vi "Dual_image_synced.vi"() -> ()   [LabVIEW 2013]
uses:
  <vilib>/DAQmx/create/channels.llb/DAQmx Create Channel (CO-Pulse Generation-Frequency).vi
  <vilib>/DAQmx/configure/timing.llb/DAQmx Timing (Implicit).vi
  <vilib>/vision/driver/NI_Vision_Acquisition_Software.lvlib
  <resource>/objmgr/imaqdx.rc
  <resource>/objmgr/daqmx.rc
panel:
  in  "Gain 2":dbl(slide)=575.0 min=350.0 max=1000.0 step=1.0 scale=350.0..1000.0
  in  "VR2":dbl(slide)=65.0 min=0.0 max=255.0 step=1.0 scale=0.0..255.0
  in  "VR1":dbl(slide)=60.0 min=0.0 max=255.0 step=1.0 scale=0.0..255.0
  in  "UB2":dbl(slide)=160.0 min=0.0 max=255.0 step=1.0 scale=0.0..255.0
  in  "UB1":dbl(slide)=165.0 min=0.0 max=255.0 step=1.0 scale=0.0..255.0
  in  "Shutter":dbl(slide)=4095.0 min=0.0 max=4095.0 step=1.0 scale=4.095..4095.0 scale format="%#.0f"
  in  "Brightness":dbl(slide)=100.0 min=0.0 max=255.0 step=1.0 scale=0.0..255.0
  in  "Gain":dbl(slide)=600.0 min=350.0 max=1000.0 step=1.0 scale=350.0..1000.0
  in  "Test Description":string="test"
  in  "Storage Directory":path=path "C:/Users/Regen/Desktop/Users/Ryan Gergely/3D_DIC"
  out "Image 2":T1(plugin-control)
  out "Buffer Number 2":u32
  out "Frame Rate 2":dbl
  in  "Camera Name 2":refnum<k21>="cam2" caption="IMAQdx Session"
  in  "Pule Frequency":dbl=2.0 format="%.1f"
  out "Actual Duty Cycle":dbl
  out "Actual Pulse Frequency":dbl
  in  "Stop":bool
  in  "Start Trigger Mode":bool
  out "Frame Rate 1":dbl
  out "Buffer Number 1":u32
  in  "Camera Name 1":refnum<k21>="cam1" caption="IMAQdx Session"
  out "Image":T1(plugin-control)
  # "1) Set Test Description and Storage Directory"
  # "2) Select Cameras"
  # "3) Start VI"
  # "4) Set Frequency and Exposure and White Balance\n(Before Start Trigger)"
  # "5)"
  # "6) Stop When Done"
  # "Exposure Settings - Both Cameras"
  # "White Balance - Camera1"
  # "White Balance - Camera2"
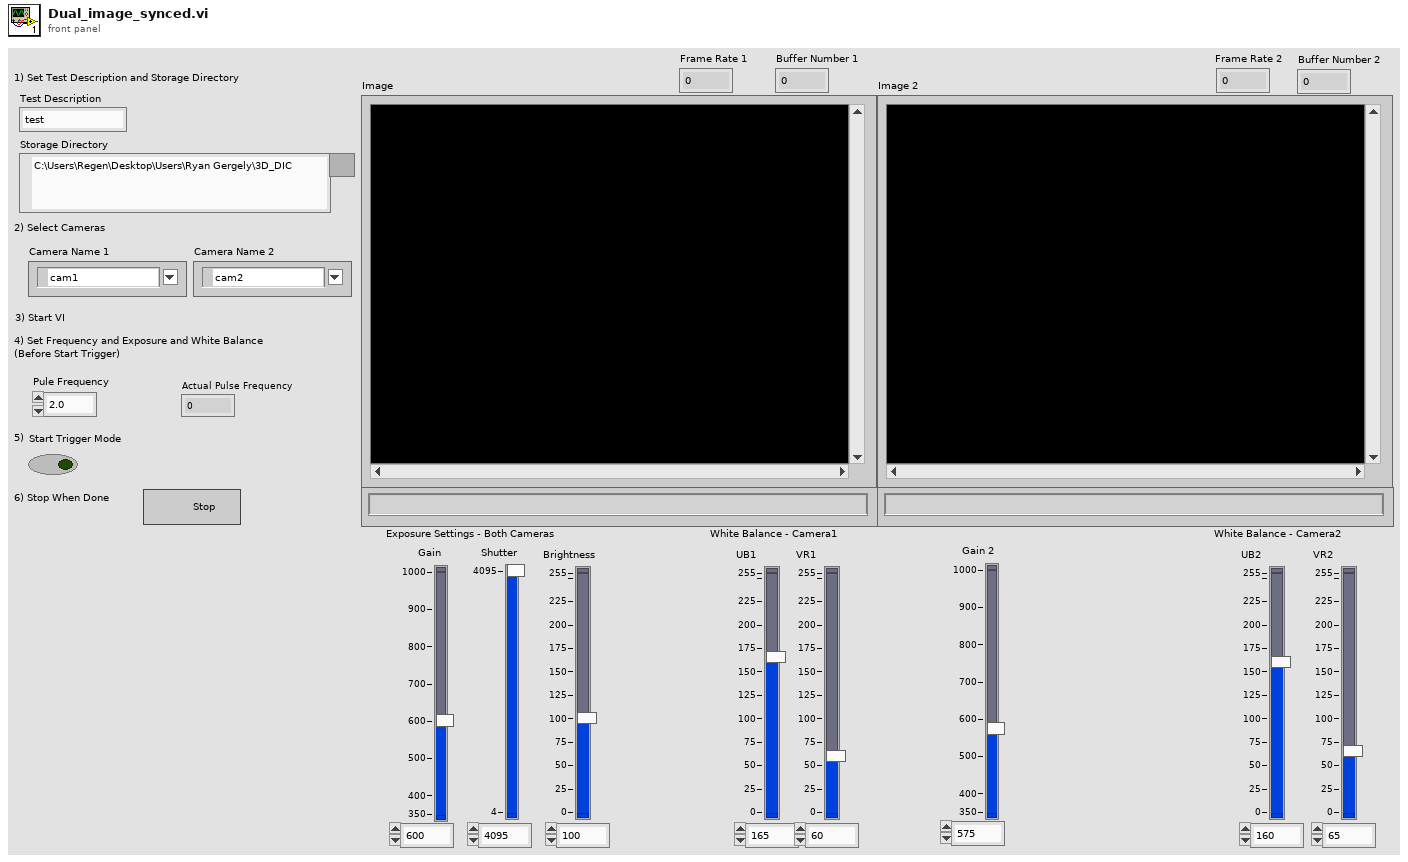
[diagram p1: front panel]
types:
  T1 = typedef "IMAQ Image.ctl" = refnum<image>
  T2 = typedef "IMAQdx.ctl" = refnum<k21>
  T3 = cluster{"Trigger Mode":u32, "Trigger Activation":u32, "Timeout (ms)":u32}
  T4 = enum16{"open", "replace", "create", "open or create", "replace or create", "replace or create with confirmation"}
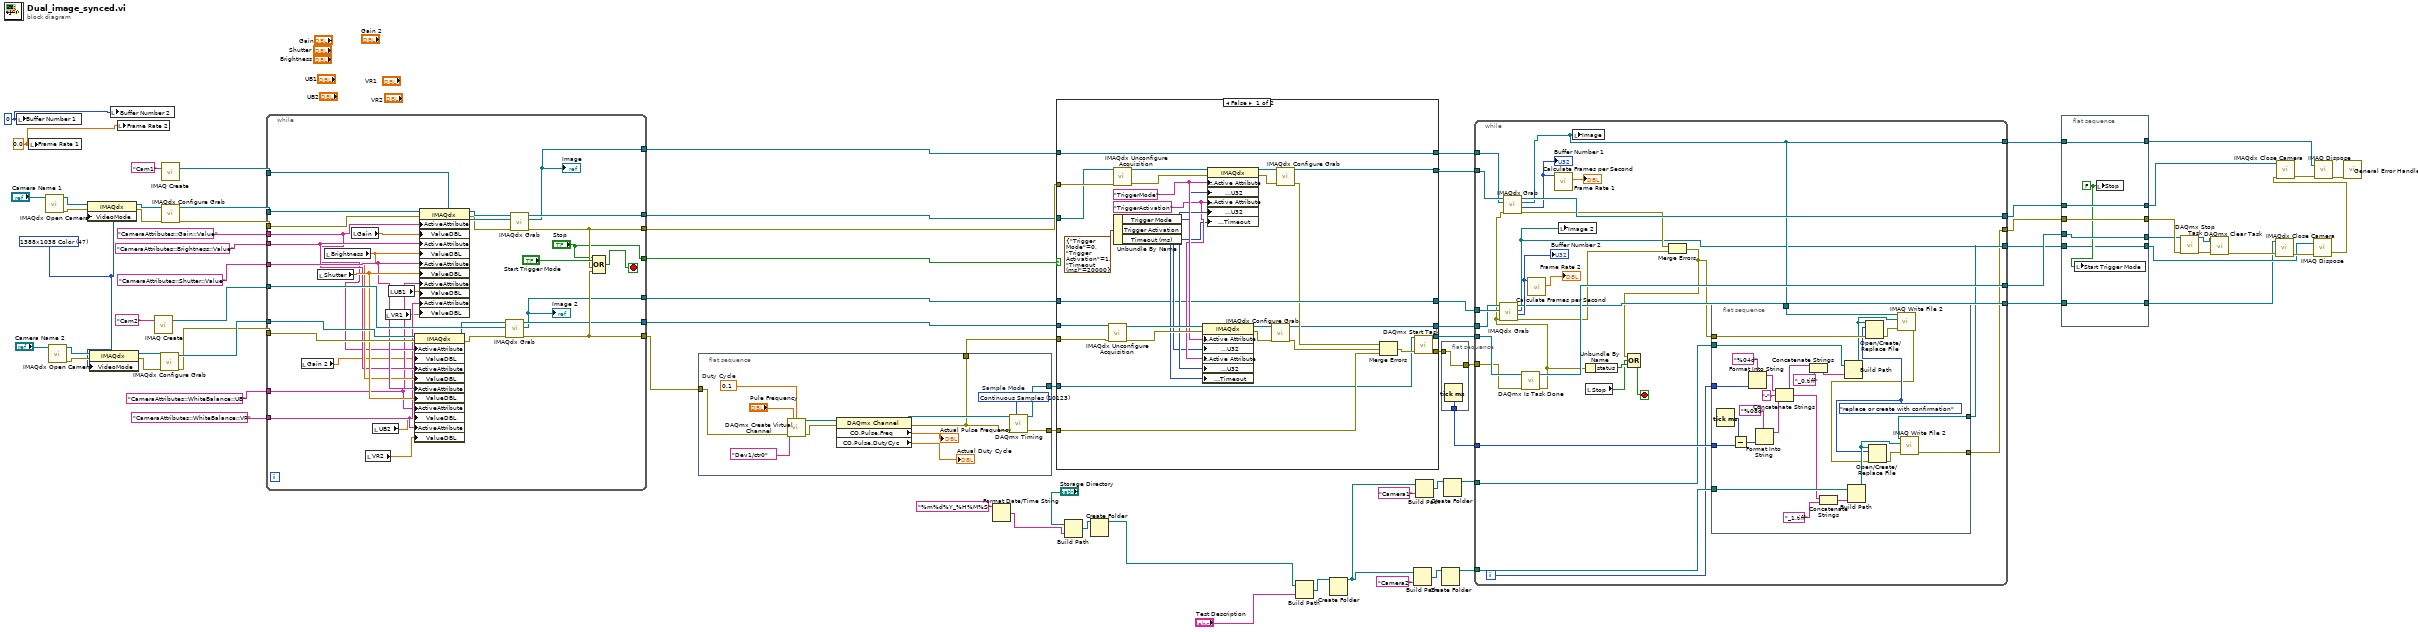
[diagram p0: block diagram]
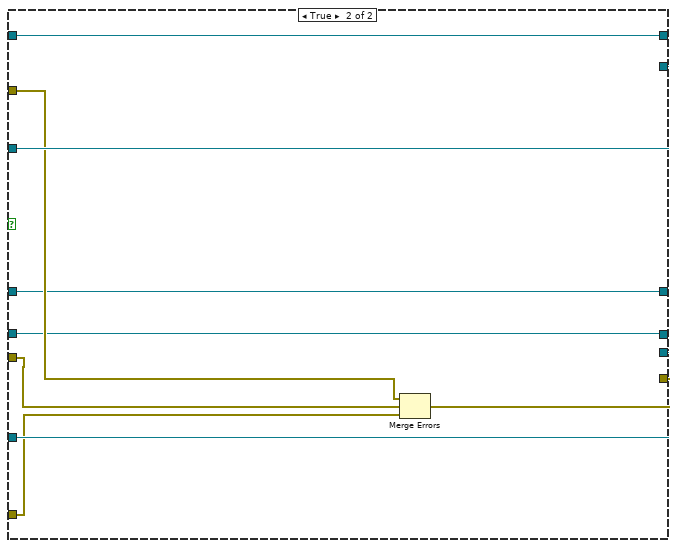
[diagram p2: hidden frame]
diagram:
  w12 = u32 47 items=["320x240 Color"=4, "640x480 Mono8"=9, "640x480 Mono16"=19, "640x480 Color"=14, "800x600 Mono8"=21, "800x600 Mono16"=27, "800x600 Color"=24, "1024x768 Mono8"=30, "1024x768 Mono16"=36, "1024x768 Color"=33, "1280x960 Mono8"=40, "1280x960 Mono16"=46, "1280x960 Color"=43, "1388x1038 Color"=47, "1388x1038 Mono"=48] ("Video Mode")
  w13 = 0.0 ("Frame Rate 1")
  w14 = u32 0 ("Buffer Number 1")
  n1 = local write "Buffer Number 1"(w14) -> ()
  n2 = local write "Frame Rate 1"(w13) -> ()
  n3 = call <vilib>:"IMAQdx Open Camera.vi"("Session In"="Camera Name 1") -> ("error out"=w20:errorcluster, "Session Out"=w22:T2)  [unwired: 2 in, 7 out]
  n4 = call <vilib>:"IMAQdx Open Camera.vi"("Session In"="Camera Name 2") -> ("error out"=w15:errorcluster, "Session Out"=w16:T2)  [unwired: 2 in, 7 out]
  n5 = property class="IMAQdx"(reference=w22, error in=w20, "VideoMode"=w12) -> (reference out=w21:T2, error out=w19:errorcluster)
  n6 = property class="IMAQdx"(reference=w16, error in=w15, "VideoMode"=w12) -> (reference out=w18:T2, error out=w17:errorcluster)
  n7 = local write "Buffer Number 2"(w14) -> ()
  n8 = local write "Frame Rate 2"(w13) -> ()
  n9 = call "IMAQ Create"("Image Name"="Cam2") -> ("New Image"=w9:T1)  [unwired: 3 in, 2 out]
  n10 = call <vilib>:"IMAQdx Configure Grab.vi"("error in"=w17, "Session In"=w18) -> ("error out"=w51:errorcluster, "Session Out"=w52:T2)  [unwired: 8 out]
  n11 = call "IMAQ Create"("Image Name"="Cam1") -> ("New Image"=w62:T1)  [unwired: 3 in, 2 out]
  n12 = call <vilib>:"IMAQdx Configure Grab.vi"("error in"=w19, "Session In"=w21) -> ("error out"=w60:errorcluster, "Session Out"=w61:T2)  [unwired: 8 out]
  n13 = while {
    tunnel: [w109] -> w73
    tunnel: w60 -> [w96]
    tunnel: w61 -> [w98]
    tunnel: [w105] -> w74
    tunnel: w62 -> [w100]
    tunnel: [w108] -> w57
    tunnel: ["Stop"] -> w58
    tunnel: w52 -> [w94]
    tunnel: w51 -> [w93]
    tunnel: [w103] -> w11
    tunnel: [w102] -> w50
    tunnel: [w101] -> w49
    tunnel: w9 -> [w99]
    tunnel: "CameraAttributes::Shutter::Value" ("ActiveAttribute") -> [w89]
    tunnel: "CameraAttributes::Brightness::Value" ("ActiveAttribute") -> [w87]
    tunnel: "CameraAttributes::Gain::Value" ("ActiveAttribute") -> [w85]
    tunnel: "CameraAttributes::WhiteBalance::UB" ("ActiveAttribute") -> [w82]
    tunnel: "CameraAttributes::WhiteBalance::VR" ("ActiveAttribute") -> [w83]
    stop <- w106 stop-if-true
    n14 = local read "Gain 2"() -> (w78:dbl)
    n15 = local read "Shutter"() -> (w90:dbl)
    n16 = local read "Brightness"() -> (w88:dbl)
    n17 = local read "Gain"() -> (w86:dbl)
    n18 = local read "VR2"() -> (w79:dbl)
    n19 = local read "UB2"() -> (w81:dbl)
    n20 = local read "VR1"() -> (w80:dbl)
    n21 = local read "UB1"() -> (w84:dbl)
    n22 = property class="IMAQdx"(reference=w94, error in=w93, "ActiveAttribute"=w85, "ValueDBL"=w78, "ActiveAttribute"=w87, "ValueDBL"=w88, "ActiveAttribute"=w89, "ValueDBL"=w90, "ActiveAttribute"=w82, "ValueDBL"=w81, "ActiveAttribute"=w83, "ValueDBL"=w79) -> (reference out=w91:T2, error out=w92:errorcluster)
    n23 = property class="IMAQdx"(reference=w98, error in=w96, "ActiveAttribute"=w85, "ValueDBL"=w86, "ActiveAttribute"=w87, "ValueDBL"=w88, "ActiveAttribute"=w89, "ValueDBL"=w90, "ActiveAttribute"=w82, "ValueDBL"=w84, "ActiveAttribute"=w83, "ValueDBL"=w80) -> (reference out=w97:T2, error out=w95:errorcluster)
    n24 = call <vilib>:"IMAQdx Grab.vi"("error in"=w92, "Image In"=w99, "Session In"=w91) -> ("error out"=w103:errorcluster, "Image Out"=w101:T1, "Session Out"=w102:T2)  [unwired: 1 in, 5 out]
    "Image 2" <- w101
    n25 = call <vilib>:"IMAQdx Grab.vi"("error in"=w95, "Image In"=w100, "Session In"=w97) -> ("error out"=w105:errorcluster, "Image Out"=w108:T1, "Session Out"=w109:T2)  [unwired: 1 in, 5 out]
    "Image" <- w108
    n26 = Compound Arithmetic op=OR("Stop", "Start Trigger Mode", w105, w103) -> (w106:bool)
  }
  n27 = flat-sequence {
    tunnel: [w113] -> w55
    tunnel: [w112] -> w48
    tunnel: w11 -> [w111]
    tunnel: [w110] -> w10
    frame #0 {
      w120 = 0.1  # Duty Cycle
      w114 = 10123 items=["Finite Samples"=10178, "Continuous Samples"=10123, "Hardware Timed Single Point"=12522]  # Sample Mode
      n28 = call-poly <vilib>:"DAQmx Create Virtual Channel.vi"("frequency"="Pule Frequency", "duty cycle"=w120, "counter"=tag "Dev1/ctr0" ("Counter"), "error in"=w111) -> ("task out"=w116:refnum<k21>, "error out"=w117:errorcluster)  [unwired: 10 in]
      n29 = property class="DAQmx Channel"(reference=w116, error in=w117) -> (reference out=w118:refnum<k21>, error out=w110:errorcluster, "CO.Pulse.Freq"=→"Actual Pulse Frequency":dbl, "CO.Pulse.DutyCyc"=→"Actual Duty Cycle":dbl)
      n30 = call-poly <vilib>:"DAQmx Timing.vi"("task/channels in"=w118, "sample mode"=w114, "error in"=w110) -> ("task out"=w113:refnum<k21>, "error out"=w112:errorcluster)  [unwired: 11 in]
    }
  }
  n31 = Format Date/Time String(time format string (%c)="%m%d%Y_%H%M%S") -> (date/time string=w34:string)  [unwired: 2 in]
  n32 = case shown="False" w58 {
    tunnel: w74 -> [w151 w157]
    tunnel: w73 -> [w150 w160]
    tunnel: [w149 w160] -> w72
    tunnel: [w130 w156] -> w3
    tunnel: [w131 w158] -> w70
    tunnel: w57 -> [w143 w159]
    tunnel: [w143 w159] -> w56
    tunnel: w55 -> [w123 w158]
    tunnel: w10 -> [w134 w155]
    tunnel: w50 -> [w133 w152]
    tunnel: w49 -> [w132 w153]
    tunnel: [w132 w153] -> w47
    tunnel: w48 -> [w126 w154]
    tunnel: [w124 w152] -> w46
    frame False {
      w137 = "TriggerActivation" ("ActiveAttribute")
      w139 = "TriggerMode" ("ActiveAttribute")
      n33 = call <vilib>:"IMAQdx Unconfigure Acquisition.vi"("error in"=w134, "Session In"=w133) -> ("error out"=w141:errorcluster, "Session Out"=w140:T2)  [unwired: 8 out]
      n34 = call <vilib>:"IMAQdx Unconfigure Acquisition.vi"("error in"=w151, "Session In"=w150) -> ("error out"=w146:errorcluster, "Session Out"=w145:T2)  [unwired: 8 out]
      n35 = Unbundle By Name(T3 {"Trigger Mode"=0, "Trigger Activation"=1, "Timeout (ms)"=20000} ("Trigger Parameters")) -> ("Trigger Mode"=w135:u32, "Trigger Activation"=w138:u32, "Timeout (ms)"=w136:u32)
      n36 = property class="IMAQdx"(reference=w140, error in=w141, "Camera Attributes:Active Attribute"=w139, "Camera Attributes:Value:U32"=w135, "Camera Attributes:Active Attribute"=w137, "Camera Attributes:Value:U32"=w138, "Acquisition Attributes:Timeout"=w136) -> (reference out=w142:T2, error out=w129:errorcluster)
      n37 = property class="IMAQdx"(reference=w145, error in=w146, "Camera Attributes:Active Attribute"=w139, "Camera Attributes:Value:U32"=w135, "Camera Attributes:Active Attribute"=w137, "Camera Attributes:Value:U32"=w138, "Acquisition Attributes:Timeout"=w136) -> (reference out=w147:T2, error out=w148:errorcluster)
      n38 = call <vilib>:"IMAQdx Configure Grab.vi"("error in"=w129, "Session In"=w142) -> ("error out"=w127:errorcluster, "Session Out"=w124:T2)  [unwired: 8 out]
      n39 = call <vilib>:"IMAQdx Configure Grab.vi"("error in"=w148, "Session In"=w147) -> ("error out"=w125:errorcluster, "Session Out"=w149:T2)  [unwired: 8 out]
      n40 = Merge Errors(w125, w127, w126) -> (w128:errorcluster)
      n41 = call <vilib>:"DAQmx Start Task.vi"("task/channels in"=w123, "error in"=w128) -> ("task out"=w131:refnum<k21>, "error out"=w130:errorcluster)  [unwired: 12 in]
    }
    frame True {
      n42 = Merge Errors(w157, w155, w154) -> (w156:errorcluster)
    }
  }
  n43 = Build Path(base path="Storage Directory", name or relative path=w34) -> (appended path=w36:path)
  n44 = Create Folder(path (use dialog)=w36) -> (created path=w31:path)  [unwired: 2 in, 2 out]
  n45 = Build Path(base path=w31, name or relative path="Test Description") -> (appended path=w30:path)
  n46 = Create Folder(path (use dialog)=w30) -> (created path=w24:path)  [unwired: 2 in, 2 out]
  n47 = Build Path(base path=w24, name or relative path="Camera2") -> (appended path=w25:path)
  n48 = Build Path(base path=w24, name or relative path="Camera1") -> (appended path=w28:path)
  n49 = flat-sequence {
    tunnel: w3 -> [w162]
    tunnel: [w162] -> w2
    tunnel: [w161] -> w1
    frame #0 {
      n50 = Tick Count (ms)() -> (millisecond timer value=w161:u32)
    }
  }
  n51 = Create Folder(path (use dialog)=w25) -> (created path=w23:path)  [unwired: 2 in, 2 out]
  n52 = Create Folder(path (use dialog)=w28) -> (created path=w27:path)  [unwired: 2 in, 2 out]
  n53 = while {
    tunnel: [w189] -> w66
    tunnel: [w167] -> w67
    tunnel: w72 -> [w186]
    tunnel: w56 -> [w185]
    tunnel: [w182] -> w68
    tunnel: w70 -> [w181]
    tunnel: w47 -> [w178]
    tunnel: w46 -> [w177]
    tunnel: w2 -> [w174]
    tunnel: [w171] -> w38
    tunnel: [w170] -> w42
    tunnel: [w173] -> w40
    tunnel: w27 -> [w164]
    tunnel: w23 -> [w172]
    tunnel: w1 -> [w166]
    i -> [w163]
    stop <- w183 stop-if-true
    n54 = call <vilib>:"DAQmx Is Task Done.vi"("task/channels in"=w181, "error in"=w174) -> ("task out"=w182:refnum<k21>, "error out"=w168:errorcluster)  [unwired: 11 in, 1 out]
    n55 = call <vilib>:"IMAQdx Grab.vi"("error in"=w168, "Image In"=w178, "Session In"=w177) -> ("error out"=w169:errorcluster, "Buffer Number Out"=w176:u32, "Image Out"=w170:T1, "Session Out"=w173:T2)  [unwired: 1 in, 4 out]
    "Buffer Number 2" <- w176
    n56 = call <vilib>:"IMAQdx Grab.vi"("error in"=w168, "Image In"=w185, "Session In"=w186) -> ("error out"=w175:errorcluster, "Buffer Number Out"=w187:u32, "Image Out"=w171:T1, "Session Out"=w189:T2)  [unwired: 1 in, 4 out]
    "Buffer Number 1" <- w187
    n57 = call <vilib>:"Calculate Frames per Second.vi"("Buffer Number"=w176) -> ("Processed Frames/s"=→"Frame Rate 2":dbl)  [unwired: 8 in, 2 out]
    n58 = call <vilib>:"Calculate Frames per Second.vi"("Buffer Number"=w187) -> ("Processed Frames/s"=→"Frame Rate 1":dbl)  [unwired: 8 in, 2 out]
    n59 = local write "Image 2"(w170) -> ()
    n60 = local write "Image"(w171) -> ()
    n61 = Unbundle By Name(w168) -> ("status"=w184:bool)
    n62 = local read "Stop"() -> (w180:bool)
    n63 = Merge Errors(w175, w169) -> (w165:errorcluster)
    n64 = Compound Arithmetic op=OR(w165, w180, w184) -> (w183:bool)
    n65 = flat-sequence {
      tunnel: w164 -> [w215]
      tunnel: w172 -> [w214]
      tunnel: w171 -> [w213]
      tunnel: w170 -> [w212]
      tunnel: w165 -> [w211]
      tunnel: [w210] -> w167
      tunnel: w166 -> [w203]
      tunnel: w163 -> [w195]
      frame #0 {
        w207 = T4."replace or create with confirmation" ("operation (0:open)")
        n66 = Tick Count (ms)() -> (millisecond timer value=w202:u32)
        n67 = Subtract(x=w202, y=w203) -> (x-y=w198:u32)
        n68 = Format Into String(format string="%04d", w195) -> (resulting string=w193:string)  [unwired: 2 in, 1 out]
        n69 = Format Into String(format string="%08d", w198) -> (resulting string=w197:string)  [unwired: 2 in, 1 out]
        n70 = Concatenate Strings(w193, "-" ("string"), w197) -> (w190:string)
        n71 = Concatenate Strings(w190, "_0.tiff") -> (w200:string)
        n72 = Concatenate Strings(w190, "_1.tiff") -> (w201:string)
        n73 = Build Path(base path=w215, name or relative path=w200) -> (appended path=w209:path)
        n74 = Build Path(base path=w214, name or relative path=w201) -> (appended path=w208:path)
        n75 = Open/Create/Replace File(file path (use dialog)=w209, error in=w211, operation (0:open)=w207) -> (error out=w206:errorcluster)  [unwired: 3 in, 2 out]
        n76 = call-poly "IMAQ Write File 2"("error in (no error)"=w206, "File Path"=w209, "Image"=w213) -> ("error out"=w204:errorcluster)  [unwired: 7 in, 1 out]
        n77 = Open/Create/Replace File(file path (use dialog)=w208, error in=w204, operation (0:open)=w207) -> (error out=w205:errorcluster)  [unwired: 3 in, 2 out]
        n78 = call-poly "IMAQ Write File 2"("error in (no error)"=w205, "File Path"=w208, "Image"=w212) -> ("error out"=w210:errorcluster)  [unwired: 7 in, 1 out]
      }
    }
  }
  n79 = flat-sequence {
    tunnel: w68 -> [w220]
    tunnel: w67 -> [w221]
    tunnel: w66 -> [w222]
    tunnel: [w222] -> w65
    tunnel: [w221] -> w64
    tunnel: [w220] -> w63
    tunnel: [w218] -> w41
    tunnel: w42 -> [w218]
    tunnel: w40 -> [w217]
    tunnel: [w217] -> w39
    tunnel: w38 -> [w216]
    tunnel: [w216] -> w37
    frame #0 {
      w219 = FALSE ("Stop")
      n80 = local write "Start Trigger Mode"(w219) -> ()
      n81 = local write "Stop"(w219) -> ()
    }
  }
  n82 = call <vilib>:"DAQmx Stop Task.vi"("task/channels in"=w63, "error in"=w64) -> ("task out"=w69:refnum<k21>, "error out"=w71:errorcluster)  [unwired: 12 in]
  n83 = call <vilib>:"DAQmx Clear Task.vi"("task in"=w69, "error in"=w71) -> ("error out"=w43:errorcluster)  [unwired: 13 in]
  n84 = call <vilib>:"IMAQdx Close Camera.vi"("error in"=w43, "Session In"=w39) -> ("error out"=w45:errorcluster)  [unwired: 9 out]
  n85 = call "IMAQ Dispose"("Image"=w41, "error in (no error)"=w45) -> ("error out"=w44:errorcluster)  [unwired: 4 in]
  n86 = call <vilib>:"IMAQdx Close Camera.vi"("error in"=w44, "Session In"=w65) -> ("error out"=w77:errorcluster)  [unwired: 9 out]
  n87 = call "IMAQ Dispose"("Image"=w37, "error in (no error)"=w77) -> ("error out"=w76:errorcluster)  [unwired: 4 in]
  n88 = call <vilib>:"General Error Handler.vi"("error in (no error)"=w76) -> ()  [unwired: 1 in, 14 out]
